vi "Enumerate Devices.vi"(8 "error in (no error)":errorcluster) -> (0 "error out":errorcluster, 3 "Devices":T1[](array[typedef]))   [LabVIEW 2020, in "devices.lvlib"]
uses:
  devices.lvlib
  Device Enumeration.ctl
  bin/gindustrialcam_32-1.dll
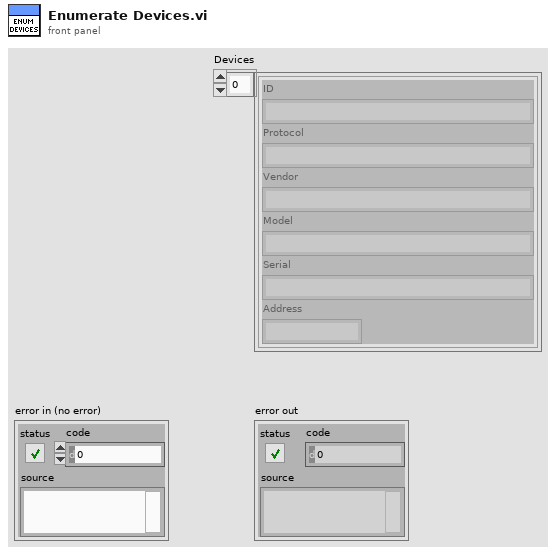
[diagram p1: front panel]
types:
  T1 = typedef "devices.lvlib/Device Enumeration.ctl" = cluster{"ID":string, "Protocol":string, "Vendor":string, "Model":string, "Serial":string, "Address":string}
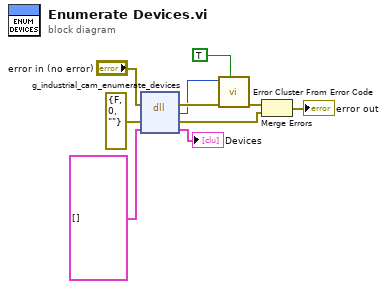
[diagram p0: block diagram]
diagram:
  n1 = dll-call lib="C:/Workspace/SSDC/g-industrial-camera/LabVIEW/bin/gindustrialcam_*-1.dll" fn="g_industrial_cam_enumerate_devices"(error in="error in (no error)", "Error"=errorcluster {"status"=FALSE, "code"=0, "source"=""} ("error constant"), "Enumeration"=T1[] [] ("Array")) -> (error out=w7:errorcluster, "MgError"=w6:i32, "Error"=w3:errorcluster, "Enumeration"=→"Devices":T1[])  [unwired: 2 in, 1 out]
  n2 = call <vilib>:"Error Cluster From Error Code.vi"("show call chain? (False)"=TRUE, "error in (no error)"=w7, "error code (0)"=w6) -> ("error out"=w4:errorcluster)  [unwired: 6 in]
  n3 = Merge Errors(w4, w3) -> (→"error out":errorcluster)
